vi "log analysis_gps.vi"() -> ()   [LabVIEW 2018] (continued)
\t1.658329\t-32.484656\t0.295000\t-0.002000\n\t\n15:23:55.0\tlog_raw\tgps_raw\t\tsystem status\tnormal 2 28.000000 0 0\trobot status\t288.054349\t67.318157\t10.021200\t0.546760\t1.689082\t-32.708365\t0.296000\t-0.003000\n\t\n15:23:55.5\tlog_raw\tgps_raw\t\tsystem status\tnormal 2 28.000000 0 0\trobot status\t288.169881\t67.229104\t10.024500\t0.591607\t1.733278\t-32.973827\t0.300000\t-0.009000\n\t\n15:23:56.1\tlog_raw\tgps_raw\t\tsystem status\tnormal 2 28.000000 0 0\trobot status\t288.285609\t67.140045\t10.028000\t0.529949\t1.703356\t-33.215106\t0.298000\t0.000000\n\t\n15:23:56.6\tlog_raw\tgps_raw\t\tsystem status\tnormal 2 28.000000 0 0\trobot status\t288.402896\t67.050197\t10.031000\t0.382545\t1.691064\t-33.405018\t0.303000\t-0.003000\n\t\n15:23:57.1\tlog_raw\tgps_raw\t\tsystem status\tnormal 2 28.100000 0 0\trobot status\t288.517996\t66.960392\t10.034600\t0.327686\t1.686813\t-33.520198\t0.306000\t0.000000\n\t\n15:23:57.6\tlog_raw\tgps_raw\t\tsystem status\tnormal 2 28.000000 0 0\trobot status\t288.617756\t66.878917\t10.037200\t0.388032\t1.762580\t-33.580696\t0.303000\t0.002000\n\t\n15:23:58.1\tlog_raw\tgps_raw\t\tsystem status\tnormal 2 28.000000 0 0\trobot status\t288.719206\t66.796540\t10.039700\t0.378367\t1.729293\t-33.611811\t0.296000\t-0.002000\n\t\n15:23:58.6\tlog_raw\tgps_raw\t\tsystem status\tnormal 2 28.000000 0 0\trobot status\t288.836366\t66.703108\t10.044100\t0.361317\t1.705497\t-33.618603\t0.298000\t0.013000\n\t\n15:23:59.1\tlog_raw\tgps_raw\t\tsystem status\tnormal 2 28.100000 0 0\trobot status\t288.954814\t66.609318\t10.047600\t0.188474\t1.632399\t-33.719352\t0.298000\t0.002000\n\t\n15:23:59.6\tlog_raw\tgps_raw\t\tsystem status\tnormal 2 28.100000 0 0\trobot status\t289.061981\t66.520928\t10.049900\t0.103210\t1.484384\t-33.752423\t0.295000\t0.002000\n\t\n15:24:00.1\tlog_raw\tgps_raw\t\tsystem status\tnormal 2 28.100000 0 0\trobot status\t289.171147\t66.430812\t10.051400\t0.015766\t1.445390\t-33.779693\t0.306000\t-0.012000\n\t\n15:24:00.6\tlog_raw\tgps_raw\t\tsystem status\tnormal 2 28.000000 0 0\trobot status\t289.280457\t66.339929\t10.054600\t-0.046571\t1.317193\t-33.648397\t0.286000\t0.023000\n\t\n15:24:01.1\tlog_raw\tgps_raw\t\tsystem status\tnormal 2 28.000000 0 0\trobot status\t289.389399\t66.249435\t10.057800\t-0.094988\t1.418269\t-33.490533\t0.253000\t0.072000\n\t\n15:24:01.6\tlog_raw\tgps_raw\t\tsystem status\tnormal 2 28.000000 0 0\trobot status\t289.499571\t66.160174\t10.062100\t-0.073967\t1.557073\t-33.178469\t0.257000\t0.075000\n\t\n15:24:02.1\tlog_raw\tgps_raw\t\tsystem status\tnormal 2 27.900000 0 0\trobot status\t289.611277\t66.070017\t10.066700\t-0.021080\t1.613738\t-32.746159\t0.225000\t0.126000\n\t\n15:24:02.6\tlog_raw\tgps_raw\t\tsystem status\tnormal 2 27.900000 0 0\trobot status\t289.725382\t65.979080\t10.070100\t-0.168702\t1.553048\t-32.226761\t0.295000\t0.028000\n\t\n15:24:03.1\tlog_raw\tgps_raw\t\tsystem status\tnormal 2 27.900000 0 0\trobot status\t289.838792\t65.888900\t10.073700\t-0.213673\t1.412012\t-31.737213\t0.429000\t-0.185000\n\t\n15:24:03.6\tlog_raw\tgps_raw\t#INSPVAXA,USB3,0,51.0,FINESTEERING,2107,282261.600,02008000,471d,15824;INS_ALIGNMENT_COMPLETE,INS_RTKFIXED,37.37072301964,126.72410864198,10.0789,22.3000,-0.1970,0.2354,0.0160,-0.160873741,1.322866529,121.119514583,0.4897,0.3148,0.6247,0.1298,0.1039,0.0767,0.1436,0.1490,5.0292,0f000001,0*85434b09\n\tsystem status\tnormal 2 27.900000 0 0\trobot status\t289.964535\t65.789209\t10.078900\t-0.160874\t1.322867\t-31.119515\t0.228000\t0.126000\n\t\n15:24:04.1\tlog_raw\tgps_raw\t#INSPVAXA,USB3,0,50.5,FINESTEERING,2107,282262.100,02008000,471d,15824;INS_ALIGNMENT_COMPLETE,INS_RTKFIXED,37.37072222272,126.72410992724,10.0823,22.3000,-0.1883,0.2369,0.0121,0.011480682,1.244674277,120.532236713,0.5693,0.3742,0.6825,0.1391,0.1098,0.0808,0.1445,0.1502,5.0254,0f000001,0*eae9fcde\n\tsystem status\tnormal 2 27.900000 0 0\trobot status\t290.078381\t65.700759\t10.082300\t0.011481\t1.244674\t-30.532237\t0.402000\t-0.130000\n\t\n15:24:04.6\tlog_raw\tgps_raw\t\tsystem status\tnormal 2 27.900000 0 0\trobot status\t290.181420\t65.629972\t10.084000\t-0.058152\t1.268255\t-30.033065\t0.380000\t-0.106000\n\t\n15:24:05.1\tlog_raw\tgps_raw\t\tsystem status\tnormal 2 27.900000 0 0\trobot status\t290.297225\t65.551573\t10.086000\t-0.219918\t1.150608\t-29.591429\t0.319000\t-0.025000\n\t\n15:24:05.6\tlog_raw\tgps_raw\t\tsystem status\tnormal 2 27.900000 0 0\trobot status\t290.413924\t65.470886\t10.089900\t-0.135917\t1.226255\t-29.162288\t0.353000\t-0.073000\n\t\n15:24:06.1\tlog_raw\tgps_raw\t\tsystem status\tnormal 2 28.000000 0 0\trobot status\t290.533106\t65.389467\t10.093600\t-0.089830\t1.183104\t-28.764617\t0.265000\t0.050000\n\t\n15:24:06.6\tlog_raw\tgps_raw\t\tsystem status\tnormal 2 28.000000 0 0\trobot status\t290.651382\t65.308209\t10.098300\t-0.148779\t1.341116\t-28.590743\t0.243000\t0.082000\n\t\n15:24:07.1\tlog_raw\tgps_raw\t\tsystem status\tnormal 2 28.000000 0 0\trobot status\t290.773116\t65.224624\t10.102200\t-0.235539\t1.356996\t-28.548470\t0.418000\t-0.171000\n\t\n15:24:07.6\tlog_raw\tgps_raw\t\tsystem status\tnormal 2 28.000000 0 0\trobot status\t290.891925\t65.142977\t10.104900\t-0.138580\t1.190893\t-28.503254\t0.342000\t-0.063000\n\t\n15:24:08.1\tlog_raw\tgps_raw\t\tsystem status\tnormal 2 28.000000 0 0\trobot status\t291.012059\t65.060352\t10.108400\t-0.108697\t1.088860\t-28.543618\t0.294000\t0.001000\n\t\n15:24:08.6\tlog_raw\tgps_raw\t#INSPVAXA,USB3,0,49.5,FINESTEERING,2107,282266.600,02000000,471d,15824;INS_ALIGNMENT_COMPLETE,INS_RTKFIXED,37.37071564001,126.72412194317,10.1142,22.3000,-0.1803,0.2485,0.0162,-0.167874326,0.987777383,118.589325472,0.4588,0.3004,0.5750,0.1240,0.0989,0.0769,0.1427,0.1481,5.0170,0f000001,0*94bf16e1\n\tsystem status\tnormal 2 28.000000 0 0\trobot status\t291.142733\t64.970143\t10.114200\t-0.167874\t0.987777\t-28.589325\t0.302000\t-0.008000\n\t\n15:24:09.1\tlog_raw\tgps_raw\t#INSPVAXA,USB3,0,51.5,FINESTEERING,2107,282267.100,02000000,471d,15824;INS_ALIGNMENT_COMPLETE,INS_RTKFIXED,37.37071488193,126.72412330620,10.1185,22.3000,-0.1782,0.2546,0.0105,-0.234897053,0.733993944,118.660329802,0.4588,0.3004,0.5750,0.1240,0.0989,0.0769,0.1427,0.1481,5.0170,0f000001,0*405246e9\n\tsystem status\tnormal 2 28.100000 0 0\trobot status\t291.263468\t64.886003\t10.118500\t-0.234897\t0.733994\t-28.660330\t0.301000\t-0.005000\n\t\n15:24:09.6\tlog_raw\tgps_raw\t\tsystem status\tnormal 2 28.100000 0 0\trobot status\t291.372920\t64.805007\t10.121900\t-0.262953\t0.652445\t-28.756882\t0.296000\t-0.023000\n\t\n15:24:10.1\tlog_raw\tgps_raw\t#INSPVAXA,USB3,0,50.5,FINESTEERING,2107,282268.100,02000000,471d,15824;INS_ALIGNMENT_COMPLETE,INS_RTKFIXED,37.37071326261,126.72412602696,10.1265,22.3000,-0.1797,0.2316,0.0106,-0.308837193,0.760008710,118.874107108,0.4588,0.3004,0.5750,0.1240,0.0989,0.0769,0.1427,0.1481,5.0170,0f000001,0*38424b3d\n\tsystem status\tnormal 2 28.100000 0 0\trobot status\t291.504468\t64.706275\t10.126500\t-0.308837\t0.760009\t-28.874107\t0.298000\t-0.019000\n\t\n15:24:10.6\tlog_raw\tgps_raw\t#INSPVAXA,USB3,0,50.5,FINESTEERING,2107,282268.600,02000000,471d,15824;INS_ALIGNMENT_COMPLETE,INS_RTKFIXED,37.37071245816,126.72412735967,10.1316,22.3000,-0.1815,0.2421,0.0127,-0.377106953,0.735852772,118.906106803,0.4588,0.3004,0.5750,0.1240,0.0989,0.0769,0.1427,0.1481,5.0170,0f000001,0*11ddd4c2\n\tsystem status\tnormal 2 28.100000 0 0\trobot status\t291.622517\t64.616989\t10.131600\t-0.377107\t0.735853\t-28.906107\t0.300000\t-0.012000\n\t\n15:24:11.1\tlog_raw\tgps_raw\t\tsystem status\tnormal 2 28.000000 0 0\trobot status\t291.731243\t64.535198\t10.136600\t-0.341882\t0.790169\t-29.060160\t0.298000\t-0.013000\n\t\n15:24:11.6\tlog_raw\tgps_raw\t#INSPVAXA,USB3,0,50.0,FINESTEERING,2107,282269.600,02000000,471d,15824;INS_ALIGNMENT_COMPLETE,INS_RTKFIXED,37.37071107493,126.72412999444,10.1387,22.3000,-0.1723,0.2314,0.0190,-0.521024846,1.079546483,119.280736819,0.5511,0.3672,0.6510,0.1337,0.1063,0.0814,0.1442,0.1496,5.0179,0f000001,0*5d398b6e\n\tsystem status\tnormal 2 28.100000 0 0\trobot status\t291.855901\t64.463464\t10.138700\t-0.521025\t1.079546\t-29.280737\t0.297000\t-0.008000\n\t\n15:24:12.1\tlog_raw\tgps_raw\t\tsystem status\tnormal 2 28.000000 0 0\trobot status\t291.955887\t64.404588\t10.140700\t-0.591155\t1.099206\t-29.528758\t0.294000\t-0.010000\n\t\n15:24:12.6\tlog_raw\tgps_raw\t#INSPVAXA,USB3,0,51.0,FINESTEERING,2107,282270.600,02008000,471d,15824;INS_ALIGNMENT_COMPLETE,INS_RTKFIXED,37.37070978971,126.72413254865,10.1460,22.3000,-0.1852,0.2381,0.0080,-0.437420088,1.249078779,119.796376349,0.5043,0.3305,0.6212,0.1261,0.1003,0.0792,0.1434,0.1486,5.0184,0f000001,0*9b5f8ba6\n\tsystem status\tnormal 2 28.000000 0 0\trobot status\t292.082149\t64.320817\t10.146000\t-0.437420\t1.249079\t-29.796376\t0.299000\t-0.013000\n\t\n15:24:13.1\tlog_raw\tgps_raw\t#INSPVAXA,USB3,0,47.5,FINESTEERING,2107,282271.100,02008000,471d,15824;INS_ALIGNMENT_COMPLETE,INS_RTKFIXED,37.37070909074,126.72413388392,10.1504,22.3000,-0.1800,0.2456,0.0054,-0.539837627,1.179431865,120.094630407,0.4787,0.3123,0.5991,0.1229,0.0985,0.0779,0.1432,0.1482,5.0193,0f000001,0*40acc907\n\tsystem status\tnormal 2 28.000000 0 0\trobot status\t292.200425\t64.243238\t10.150400\t-0.539838\t1.179432\t-30.094630\t0.297000\t-0.007000\n\t\n15:24:13.6\tlog_raw\tgps_raw\t#INSPVAXA,USB3,0,47.5,FINESTEERING,2107,282271.600,02008000,471d,15824;INS_ALIGNMENT_COMPLETE,INS_RTKFIXED,37.37070834780,126.72413522387,10.1531,22.3000,-0.1652,0.2443,0.0195,-0.572032410,1.056169102,120.353350938,0.4787,0.3123,0.5991,0.1229,0.0985,0.0779,0.1432,0.1482,5.0193,0f000001,0*1c071485\n\tsystem status\tnormal 2 28.000000 0 0\trobot status\t292.319115\t64.160778\t10.153100\t-0.572032\t1.056169\t-30.353351\t0.301000\t-0.020000\n\t\n15:24:14.1\tlog_raw\tgps_raw\t\tsystem status\tnormal 2 28.100000 0 0\trobot status\t292.425435\t64.085765\t10.154600\t-0.607784\t0.913539\t-30.523777\t0.299000\t-0.016000\n\t\n15:24:14.6\tlog_raw\tgps_raw\t#INSPVAXA,USB3,0,48.5,FINESTEERING,2107,282272.600,02008000,471d,15824;INS_ALIGNMENT_COMPLETE,INS_RTKFIXED,37.37070676202,126.72413789177,10.1597,22.3000,-0.1767,0.2382,0.0118,-0.374820510,0.656096150,120.799348362,0.4787,0.3123,0.5991,0.1229,0.0985,0.0779,0.1432,0.1482,5.0193,0f000001,0*9be2d9dc\n\tsystem status\tnormal 2 28.100000 0 0\trobot status\t292.555434\t63.984773\t10.159700\t-0.374821\t0.656096\t-30.799348\t0.293000\t-0.014000\n\t\n15:24:15.1\tlog_raw\tgps_raw\t\tsystem status\tnormal 2 28.000000 0 0\trobot status\t292.661239\t63.902459\t10.165100\t-0.316516\t0.670151\t-31.045836\t0.294000\t-0.010000\n\t\n15:24:15.6\tlog_raw\tgps_raw\t#INSPVAXA,USB3,0,51.5,FINESTEERING,2107,282273.600,02008000,471d,15824;INS_ALIGNMENT_COMPLETE,INS_RTKFIXED,37.37070511778,126.72414055042,10.1715,22.3000,-0.1870,0.2363,0.0134,-0.459769985,0.798437213,121.336357877,0.4787,0.3123,0.5991,0.1229,0.0985,0.0779,0.1432,0.1482,5.0193,0f000001,0*703348aa\n\tsystem status\tnormal 2 28.000000 0 0\trobot status\t292.790932\t63.802279\t10.171500\t-0.459770\t0.798437\t-31.336358\t0.297000\t-0.009000\n\t\n15:24:16.1\tlog_raw\tgps_raw\t\tsystem status\tnormal 2 28.100000 0 0\trobot status\t292.895056\t63.721026\t10.176300\t-0.551373\t0.887898\t-31.600267\t0.298000\t-0.009000\n\t\n15:24:16.6\tlog_raw\tgps_raw\t#INSPVAXA,USB3,0,50.0,FINESTEERING,2107,282274.600,02000000,471d,15824;INS_ALIGNMENT_COMPLETE,INS_RTKFIXED,37.37070363879,126.72414308570,10.1749,22.3000,-0.1813,0.2312,0.0078,-0.604469553,1.084486216,121.923542581,0.5575,0.3692,0.6704,0.1333,0.1077,0.0814,0.1446,0.1496,5.0225,0f000001,0*5c099128\n\tsystem status\tnormal 2 28.100000 0 0\trobot status\t293.015503\t63.638127\t10.174900\t-0.604470\t1.084486\t-31.923543\t0.297000\t-0.006000\n\t\n15:24:17.1\tlog_raw\tgps_raw\t#INSPVAXA,USB3,0,50.5,FINESTEERING,2107,282275.100,02000000,471d,15824;INS_ALIGNMENT_COMPLETE,INS_RTKFIXED,37.37070296140,126.72414429321,10.1745,22.3000,-0.1748,0.2312,0.0107,-0.634765121,1.047187447,122.187120855,0.5046,0.3310,0.6337,0.1261,0.1021,0.0787,0.1438,0.1486,5.0224,0f000001,0*d0387721\n\tsystem status\tnormal 2 28.100000 0 0\trobot status\t293.122463\t63.562943\t10.174500\t-0.634765\t1.047187\t-32.187121\t0.299000\t-0.006000\n\t\n15:24:17.6\tlog_raw\tgps_raw\t#INSPVAXA,USB3,0,50.5,FINESTEERING,2107,282275.600,02000000,471d,15824;INS_ALIGNMENT_COMPLETE,INS_RTKFIXED,37.37070222382,126.72414554188,10.1759,22.3000,-0.1770,0.2216,0.0167,-0.613341338,0.949181726,122.390549431,0.5046,0.3310,0.6337,0.1261,0.1021,0.0787,0.1438,0.1486,5.0224,0f000001,0*c2bde323\n\tsystem status\tnormal 2 28.000000 0 0\trobot status\t293.233068\t63.481079\t10.175900\t-0.613341\t0.949182\t-32.390549\t0.296000\t-0.002000\n\t\n15:24:18.1\tlog_raw\tgps_raw\t#INSPVAXA,USB3,0,49.0,FINESTEERING,2107,282276.100,02000000,471d,15824;INS_ALIGNMENT_COMPLETE,INS_RTKFIXED,37.37070146570,126.72414680907,10.1773,22.3000,-0.1774,0.2243,0.0157,-0.609174519,0.899706635,122.569585175,0.4767,0.3125,0.6072,0.1235,0.1004,0.0773,0.1434,0.1482,5.0223,0f000001,0*a35fb81b\n\tsystem status\tnormal 2 28.100000 0 0\trobot status\t293.345313\t63.396935\t10.177300\t-0.609175\t0.899707\t-32.569585\t0.299000\t0.000000\n\t\n15:24:18.6\tlog_raw\tgps_raw\t\tsystem status\tnormal 2 28.100000 0 0\trobot status\t293.444232\t63.320197\t10.180300\t-0.593656\t0.818984\t-32.795506\t0.301000\t-0.003000\n\t\n15:24:19.1\tlog_raw\tgps_raw\t#INSPVAXA,USB3,0,50.0,FINESTEERING,2107,282277.100,02000000,471d,15824;INS_ALIGNMENT_COMPLETE,INS_RTKFIXED,37.37069991504,126.72414929974,10.1840,22.3000,-0.1767,0.2226,0.0047,-0.557997930,0.665249909,123.001928540,0.4767,0.3125,0.6072,0.1235,0.1004,0.0773,0.1434,0.1482,5.0223,0f000001,0*cb3103e7\n\tsystem status\tnormal 2 28.100000 0 0\trobot status\t293.565933\t63.224828\t10.184000\t-0.557998\t0.665250\t-33.001929\t0.296000\t0.002000\n\t\n15:24:19.6\tlog_raw\tgps_raw\t\tsystem status\tnormal 2 28.100000 0 0\trobot status\t293.665372\t63.142839\t10.189000\t-0.617323\t0.688216\t-33.148551\t0.293000\t0.009000\n\t\n15:24:20.1\tlog_raw\tgps_raw\t#INSPVAXA,USB3,0,53.0,FINESTEERING,2107,282278.100,02000000,471d,15824;INS_ALIGNMENT_COMPLETE,INS_RTKFIXED,37.37069823681,126.72415183772,10.1961,22.3000,-0.1823,0.2204,0.0074,-0.523658025,0.566082067,123.287197308,0.4767,0.3125,0.6072,0.1235,0.1004,0.0773,0.1434,0.1482,5.0223,0f000001,0*25d51a4b\n\tsystem status\tnormal 2 28.100000 0 0\trobot status\t293.790743\t63.038563\t10.196100\t-0.523658\t0.566082\t-33.287197\t0.303000\t-0.002000\n\t\n15:24:20.6\tlog_raw\tgps_raw\t\tsystem status\tnormal 2 28.100000 0 0\trobot status\t293.892481\t62.953714\t10.201200\t-0.497645\t0.480961\t-33.302974\t0.300000\t0.011000\n\t\n15:24:21.1\tlog_raw\tgps_raw\t\tsystem status\tnormal 2 28.100000 0 0\trobot status\t294.010445\t62.857710\t10.205900\t-0.584538\t0.459280\t-33.393453\t0.299000\t0.008000\n\t\n15:24:21.6\tlog_raw\tgps_raw\t\tsystem status\tnormal 2 28.100000 0 0\trobot status\t294.125019\t62.772862\t10.206400\t-0.680267\t0.496944\t-33.443344\t0.303000\t0.004000\n\t\n15:24:22.1\tlog_raw\tgps_raw\t#INSPVAXA,USB3,0,47.5,FINESTEERING,2107,282280.100,02000000,471d,15824;INS_ALIGNMENT_COMPLETE,INS_RTKFIXED,37.37069498335,126.72415703248,10.2090,22.3000,-0.1979,0.2492,0.0153,-0.691574925,0.436072461,123.457665548,0.5547,0.3701,0.6738,0.1343,0.1087,0.0808,0.1445,0.1496,5.0239,0f000001,0*1cc0a1a6\n\tsystem status\tnormal 2 28.100000 0 0\trobot status\t294.250886\t62.677463\t10.209000\t-0.691575\t0.436072\t-33.457666\t0.308000\t0.006000\n\t\n15:24:22.6\tlog_raw\tgps_raw\t\tsystem status\tnormal 2 28.000000 0 0\trobot status\t294.357425\t62.588733\t10.214300\t-0.468577\t0.095903\t-33.413871\t0.285000\t0.024000\n\t\n15:24:23.1\tlog_raw\tgps_raw\t#INSPVAXA,USB3,0,49.5,FINESTEERING,2107,282281.100,02000000,471d,15824;INS_ALIGNMENT_COMPLETE,INS_RTKFIXED,37.37069324003,126.72415967576,10.2193,22.3000,-0.1883,0.2410,0.0110,-0.444587067,-0.239892052,123.232720595,0.5547,0.3701,0.6738,0.1343,0.1087,0.0808,0.1445,0.1496,5.0239,0f000001,0*fc1f5c5f\n\tsystem status\tnormal 2 28.000000 0 0\trobot status\t294.485024\t62.483973\t10.219300\t-0.444587\t-0.239892\t-33.232721\t0.336000\t-0.039000\n\t\n15:24:23.6\tlog_raw\tgps_raw\t\tsystem status\tnormal 2 28.000000 0 0\trobot status\t294.590664\t62.401031\t10.222200\t-0.677387\t-0.510813\t-32.931277\t0.345000\t-0.055000\n\t\n15:24:24.1\tlog_raw\tgps_raw\t#INSPVAXA,USB3,0,47.5,FINESTEERING,2107,282282.100,02000000,471d,15824;INS_ALIGNMENT_COMPLETE,INS_RTKFIXED,37.37069160850,126.72416229361,10.2264,22.3000,-0.1858,0.2281,-0.0001,-0.736056303,-0.906540815,122.497361054,0.5875,0.3887,0.7203,0.1380,0.1105,0.0818,0.1447,0.1498,5.0279,0f000001,0*0c5128b7\n\tsystem status\tnormal 2 28.000000 0 0\trobot status\t294.716909\t62.302890\t10.226400\t-0.736056\t-0.906541\t-32.497361\t0.314000\t-0.011000\n\t\n15:24:24.6\tlog_raw\tgps_raw\t#INSPVAXA,USB3,0,47.5,FINESTEERING,2107,282282.600,02000000,471d,15824;INS_ALIGNMENT_COMPLETE,INS_RTKFIXED,37.37069089697,126.72416351730,10.2196,22.3000,-0.1871,0.2326,0.0042,-0.425257190,-0.862348838,121.960644857,0.5875,0.3887,0.7203,0.1380,0.1105,0.0818,0.1447,0.1498,5.0279,0f000001,0*490a0fa5\n\tsystem status\tnormal 2 27.900000 0 0\trobot status\t294.825301\t62.223917\t10.219600\t-0.425257\t-0.862349\t-31.960645\t0.346000\t-0.056000\n\t\n15:24:25.1\tlog_raw\tgps_raw\t\tsystem status\tnormal 2 27.900000 0 0\trobot status\t294.924203\t62.153574\t10.212800\t-0.190843\t-0.823864\t-31.404317\t0.359000\t-0.071000\n\t\n15:24:25.6\tlog_raw\tgps_raw\t#INSPVAXA,USB3,0,46.5,FINESTEERING,2107,282283.600,02008000,471d,15824;INS_ALIGNMENT_COMPLETE,INS_RTKFIXED,37.37068940958,126.72416607579,10.2138,22.3000,-0.1636,0.2189,-0.0003,-0.120036604,-0.860841459,120.892387916,0.5875,0.3887,0.7203,0.1380,0.1105,0.0818,0.1447,0.1498,5.0279,0f000001,0*9192f1a2\n\tsystem status\tnormal 2 27.900000 0 0\trobot status\t295.051928\t62.058832\t10.213800\t-0.120037\t-0.860841\t-30.892388\t0.401000\t-0.149000\n\t\n15:24:26.1\tlog_raw\tgps_raw\t#INSPVAXA,USB3,0,51.5,FINESTEERING,2107,282284.100,02008000,471d,15824;INS_ALIGNMENT_COMPLETE,INS_RTKFIXED,37.37068864878,126.72416738015,10.2177,22.3000,-0.1641,0.2313,0.0038,-0.033754752,-0.589658100,120.436095799,0.5875,0.3887,0.7203,0.1380,0.1105,0.0818,0.1447,0.1498,5.0279,0f000001,0*0148cd2e\n\tsystem status\tnormal 2 27.900000 0 0\trobot status\t295.167466\t61.974391\t10.217700\t-0.033755\t-0.589658\t-30.436096\t0.215000\t0.132000\n\t\n15:24:26.6\tlog_raw\tgps_raw\t#INSPVAXA,USB3,0,51.5,FINESTEERING,2107,282284.600,02008000,471d,15824;INS_ALIGNMENT_COMPLETE,INS_RTKFIXED,37.37068791248,126.72416871170,10.2207,22.3000,-0.1613,0.2366,0.0105,-0.227472838,-0.490349868,119.960742273,0.5875,0.3887,0.7203,0.1380,0.1105,0.0818,0.1447,0.1498,5.0279,0f000001,0*af559696\n\tsystem status\tnormal 2 27.900000 0 0\trobot status\t295.285413\t61.892668\t10.220700\t-0.227473\t-0.490350\t-29.960742\t0.213000\t0.142000\n\t\n15:24:27.1\tlog_raw\tgps_raw\t#INSPVAXA,USB3,0,51.5,FINESTEERING,2107,282285.100,02008000,471d,15824;INS_ALIGNMENT_COMPLETE,INS_RTKFIXED,37.37068720846,126.72417000092,10.2252,22.3000,-0.1602,0.2440,0.0066,-0.187971792,0.385088793,119.635511852,0.5949,0.3921,0.7470,0.1392,0.1132,0.0817,0.1449,0.1501,5.0298,0f000001,0*026b0f4f\n\tsystem status\tnormal 2 27.900000 0 0\trobot status\t295.399609\t61.814529\t10.225200\t-0.187972\t0.385089\t-29.635512\t0.333000\t-0.021000\n\t\n15:24:27.6\tlog_raw\tgps_raw\t#INSPVAXA,USB3,0,52.0,FINESTEERING,2107,282285.600,02008000,471d,15824;INS_ALIGNMENT_COMPLETE,INS_RTKFIXED,37.37068652184,126.72417128801,10.2137,22.3000,-0.1658,0.2472,-0.0117,-0.055492896,0.657869792,119.429156162,0.5949,0.3921,0.7470,0.1392,0.1132,0.0817,0.1449,0.1501,5.0298,0f000001,0*cfd09dcb\n\tsystem status\tnormal 2 28.000000 0 0\trobot status\t295.513618\t61.738321\t10.213700\t-0.055493\t0.657870\t-29.429156\t0.222000\t0.118000\n\t\n15:24:28.1\tlog_raw\tgps_raw\t#INSPVAXA,USB3,0,48.5,FINESTEERING,2107,282286.100,02008000,471d,15824;INS_ALIGNMENT_COMPLETE,INS_RTKFIXED,37.37068585553,126.72417255759,10.2052,22.3000,-0.1551,0.2284,0.0107,-0.089152312,0.639970928,119.250576511,0.5190,0.3392,0.6809,0.1320,0.1082,0.0780,0.1441,0.1491,5.0307,0f000001,0*ec53885d\n\tsystem status\tnormal 2 28.000000 0 0\trobot status\t295.626075\t61.664367\t10.205200\t-0.089152\t0.639971\t-29.250577\t0.247000\t0.053000\n\t\n15:24:28.6\tlog_raw\tgps_raw\t#INSPVAXA,USB3,0,48.5,FINESTEERING,2107,282286.600,02008000,471d,15824;INS_ALIGNMENT_COMPLETE,INS_RTKFIXED,37.37068514150,126.72417389818,10.2001,22.3000,-0.1412,0.2197,0.0066,0.024364093,0.832001131,119.298455875,0.5190,0.3392,0.6809,0.1320,0.1082,0.0780,0.1441,0.1491,5.0307,0f000001,0*de9bf723\n\tsystem status\tnormal 2 28.100000 0 0\trobot status\t295.744822\t61.585116\t10.200100\t0.024364\t0.832001\t-29.298456\t0.272000\t0.056000\n\t\n15:24:29.1\tlog_raw\tgps_raw\t#INSPVAXA,USB3,0,48.5,FINESTEERING,2107,282287.100,02008000,471d,15824;INS_ALIGNMENT_COMPLETE,INS_RTKFIXED,37.37068448744,126.72417519191,10.1977,22.3000,-0.1331,0.1859,0.0151,-0.327488179,0.840633219,119.294501197,0.4827,0.3161,0.6365,0.1297,0.1073,0.0763,0.1436,0.1487,5.0297,0f000001,0*ec0356ba\n\tsystem status\tnormal 2 28.100000 0 0\trobot status\t295.859419\t61.512521\t10.197700\t-0.327488\t0.840633\t-29.294501\t0.273000\t-0.012000\n\t\n15:24:29.6\tlog_raw\tgps_raw\t#INSPVAXA,USB3,0,49.5,FINESTEERING,2107,282287.600,02000000,471d,15824;INS_ALIGNMENT_COMPLETE,INS_RTKFIXED,37.37068376486,126.72417656780,10.2009,22.3000,-0.1622,0.2304,0.0144,-0.264314636,1.151154189,119.357397918,0.4827,0.3161,0.6365,0.1297,0.1073,0.0763,0.1436,0.1487,5.0297,0f000001,0*1ac61951\n\tsystem status\tnormal 2 28.000000 0 0\trobot status\t295.981293\t61.432322\t10.200900\t-0.264315\t1.151154\t-29.357398\t0.309000\t0.000000\n\t\n15:24:30.1\tlog_raw\tgps_raw\t#INSPVAXA,USB3,0,52.0,FINESTEERING,2107,282288.100,02000000,471d,15824;INS_ALIGNMENT_COMPLETE,INS_RTKFIXED,37.37068313188,126.72417778864,10.2013,22.3000,-0.1464,0.2451,0.0101,-0.437974736,2.271326824,119.414001695,0.4827,0.3161,0.6365,0.1297,0.1073,0.0763,0.1436,0.1487,5.0297,0f000001,0*f8a30918\n\tsystem status\tnormal 2 28.000000 0 0\trobot status\t296.089433\t61.362067\t10.201300\t-0.437975\t2.271327\t-29.414002\t0.304000\t-0.003000\n\t\n15:24:30.6\tlog_raw\tgps_raw\t#INSPVAXA,USB3,0,52.0,FINESTEERING,2107,282288.600,02000000,471d,15824;INS_ALIGNMENT_COMPLETE,INS_RTKFIXED,37.37068248207,126.72417903271,10.2071,22.3000,-0.1554,0.2479,0.0102,-0.520482478,3.090095843,119.464562963,0.4827,0.3161,0.6365,0.1297,0.1073,0.0763,0.1436,0.1487,5.0297,0f000001,0*4436d63b\n\tsystem status\tnormal 2 28.000000 0 0\trobot status\t296.199631\t61.289944\t10.207100\t-0.520482\t3.090096\t-29.464563\t0.306000\t-0.003000\n\t\n15:24:31.1\tlog_raw\tgps_raw\t#INSPVAXA,USB3,0,48.0,FINESTEERING,2107,282289.100,02000000,471d,15824;INS_ALIGNMENT_COMPLETE,INS_RTKFIXED,37.37068179402,126.72418031784,10.2124,22.3000,-0.1466,0.2345,0.0076,-0.435594765,3.881928783,119.627439178,0.5155,0.3438,0.6451,0.1390,0.1110,0.0782,0.1436,0.1489,5.0203,0f000001,0*d705b298\n\tsystem status\tnormal 2 28.000000 0 0\trobot status\t296.313465\t61.213577\t10.212400\t-0.435595\t3.881929\t-29.627439\t0.294000\t-0.019000\n\t\n15:24:31.6\tlog_raw\tgps_raw\t#INSPVAXA,USB3,0,48.0,FINESTEERING,2107,282289.600,02000000,471d,15824;INS_ALIGNMENT_COMPLETE,INS_RTKFIXED,37.37068106233,126.72418156036,10.2167,22.3000,-0.1573,0.2453,0.0197,-0.196955820,4.346907241,119.830177459,0.5155,0.3438,0.6451,0.1390,0.1110,0.0782,0.1436,0.1489,5.0203,0f000001,0*c638875e\n\tsystem status\tnormal 2 28.000000 0 0\trobot status\t296.423526\t61.132367\t10.216700\t-0.196956\t4.346907\t-29.830177\t0.300000\t-0.016000\n\t\n15:24:32.1\tlog_raw\tgps_raw\t#INSPVAXA,USB3,0,45.0,FINESTEERING,2107,282290.100,02000000,471d,15824;INS_ALIGNMENT_COMPLETE,INS_RTKFIXED,37.37068031183,126.72418287504,10.2233,22.3000,-0.1663,0.2481,0.0180,-0.098835981,4.376797831,120.158403122,0.5155,0.3438,0.6451,0.1390,0.1110,0.0782,0.1436,0.1489,5.0203,0f000001,0*f931a41f\n\tsystem status\tnormal 2 28.000000 0 0\trobot status\t296.539978\t61.049069\t10.223300\t-0.098836\t4.376798\t-30.158403\t0.298000\t-0.016000\n\t\n15:24:32.6\tlog_raw\tgps_raw\t#INSPVAXA,USB3,0,45.0,FINESTEERING,2107,282290.600,02000000,471d,15824;INS_ALIGNMENT_COMPLETE,INS_RTKFIXED,37.37067956238,126.72418428483,10.2337,22.3000,-0.1707,0.2482,0.0265,-0.202932482,4.159469739,120.506147685,0.5155,0.3438,0.6451,0.1390,0.1110,0.0782,0.1436,0.1489,5.0203,0f000001,0*908c714d\n\tsystem status\tnormal 2 28.000000 0 0\trobot status\t296.664855\t60.965887\t10.233700\t-0.202932\t4.159470\t-30.506148\t0.300000\t-0.025000\n\t\n15:24:33.1\tlog_raw\tgps_raw\t#INSPVAXA,USB3,0,45.0,FINESTEERING,2107,282291.100,02000000,471d,15824;INS_ALIGNMENT_COMPLETE,INS_RTKFIXED,37.37067879937,126.72418567734,10.2444,22.3000,-0.1651,0.2543,0.0207,-0.251060851,3.844476935,120.878401990,0.5409,0.3575,0.6537,0.1355,0.1073,0.0795,0.1434,0.1485,4.9849,0f000001,0*d6642fae\n\tsystem status\tnormal 2 28.000000 0 0\trobot status\t296.788201\t60.881200\t10.244400\t-0.251061\t3.844477\t-30.878402\t0.299000\t-0.019000\n\t\n15:24:33.6\tlog_raw\tgps_raw\t#INSPVAXA,USB3,0,49.0,FINESTEERING,2107,282291.600,02000000,471d,15824;INS_ALIGNMENT_COMPLETE,INS_RTKFIXED,37.37067799408,126.72418700521,10.2537,22.3000,-0.1763,0.2581,0.0156,-0.182414041,3.404030284,121.216304080,0.5409,0.3575,0.6537,0.1355,0.1073,0.0795,0.1434,0.1485,4.9849,0f000001,0*0bbc7934\n\tsystem status\tnormal 2 28.000000 0 0\trobot status\t296.905822\t60.791821\t10.253700\t-0.182414\t3.404030\t-31.216304\t0.300000\t-0.019000\n\t\n15:24:34.1\tlog_raw\tgps_raw\t#INSPVAXA,USB3,0,45.5,FINESTEERING,2107,282292.100,02000000,471d,15824;INS_ALIGNMENT_COMPLETE,INS_RTKFIXED,37.37067717574,126.72418831770,10.2613,22.3000,-0.1798,0.2515,0.0164,-0.016177386,3.020104731,121.543147805,0.5007,0.3269,0.6199,0.1278,0.1011,0.0781,0.1427,0.1475,4.9679,0f000001,0*266eeccf\n\tsystem status\tnormal 2 28.000000 0 0\trobot status\t297.022080\t60.700994\t10.261300\t-0.016177\t3.020105\t-31.543148\t0.290000\t-0.026000\n\t\n15:24:34.6\tlog_raw\tgps_raw\t#INSPVAXA,USB3,0,45.5,FINESTEERING,2107,282292.600,02000000,471d,15824;INS_ALIGNMENT_COMPLETE,INS_RTKFIXED,37.37067636900,126.72418961762,10.2690,22.3000,-0.1769,0.2534,0.0080,-0.042843128,2.826759878,121.907768191,0.5007,0.3269,0.6199,0.1278,0.1011,0.0781,0.1427,0.1475,4.9679,0f000001,0*aaae4f23\n\tsystem status\tnormal 2 28.000000 0 0\trobot status\t297.137225\t60.611454\t10.269000\t-0.042843\t2.826760\t-31.907768\t0.292000\t-0.018000\n\t\n15:24:35.1\tlog_raw\tgps_raw\t#INSPVAXA,USB3,0,45.5,FINESTEERING,2107,282293.100,02000000,471d,15824;INS_ALIGNMENT_COMPLETE,INS_RTKFIXED,37.37067553892,126.72419093232,10.2760,22.3000,-0.1811,0.2495,0.0116,-0.008430473,2.413814082,122.277222921,0.4766,0.3108,0.5954,0.1241,0.0990,0.0774,0.1425,0.1470,4.9617,0f000001,0*c888aeda\n\tsystem status\tnormal 2 28.000000 0 0\trobot status\t297.253679\t60.519324\t10.276000\t-0.008430\t2.413814\t-32.277223\t0.308000\t-0.003000\n\t\n15:24:35.6\tlog_raw\tgps_raw\t#INSPVAXA,USB3,0,46.5,FINESTEERING,2107,282293.600,02000000,471d,15824;INS_ALIGNMENT_COMPLETE,INS_RTKFIXED,37.37067472793,126.72419224415,10.2820,22.3000,-0.1803,0.2324,0.0113,-0.180884788,2.125088791,122.585479065,0.4766,0.3108,0.5954,0.1241,0.0990,0.0774,0.1425,0.1470,4.9617,0f000001,0*8a54f30e\n\tsystem status\tnormal 2 28.000000 0 0\trobot status\t297.369878\t60.429312\t10.282000\t-0.180885\t2.125089\t-32.585479\t0.274000\t-0.042000\n\t\n15:24:36.1\tlog_raw\tgps_raw\t#INSPVAXA,USB3,0,46.5,FINESTEERING,2107,282294.100,02008000,471d,15824;INS_ALIGNMENT_COMPLETE,INS_RTKFIXED,37.37067392240,126.72419354245,10.2863,22.3000,-0.1909,0.2309,0.0096,-0.404437997,1.924119291,122.825127987,0.4614,0.3022,0.5776,0.1224,0.0977,0.0772,0.1423,0.1468,4.9609,0f000001,0*f2faedc4\n\tsystem status\tnormal 2 28.000000 0 0\trobot status\t297.484880\t60.339907\t10.286300\t-0.404438\t1.924119\t-32.825128\t0.293000\t-0.008000\n\t\n15:24:36.6\tlog_raw\tgps_raw\t#DUALANTENNAHEADINGA,USB3,0,47.0,FINESTEERING,2107,282294.600,02008000,d426,15824;SOL_COMPUTED,NARROW_FLOAT,-1.000000000,121.189437866,-60.258087158,0.0,360.000000000,180.000000000,\"631T\",18,7,7,5,04,00,20,03*d581effc\n\tsystem status\tnormal 2 28.100000 0 0\trobot status\t297.596477\t60.250156\t10.290000\t-0.474567\t1.563892\t-33.134759\t0.291000\t0.000000\n\t\n15:24:37.1\tlog_raw\tgps_raw\t#DUALANTENNAHEADINGA,USB3,0,45.0,FINESTEERING,2107,282295.100,02008000,d426,15824;SOL_COMPUTED,L1_FLOAT,-1.000000000,102.362266541,-42.452087402,0.0,360.000000000,180.000000000,\"631T\",17,6,6,3,04,00,20,01*c6a3d1e1\n\tsystem status\tnormal 2 28.000000 0 0\trobot status\t297.709107\t60.159225\t10.294100\t-0.608566\t1.421142\t-33.394057\t0.298000\t-0.001000\n\t\n15:24:37.6\tlog_raw\tgps_raw\t#DUALANTENNAHEADINGA,USB3,0,45.0,FINESTEERING,2107,282295.600,02008000,d426,15824;SOL_COMPUTED,L1_FLOAT,-1.000000000,103.041458130,-42.702667236,0.0,360.000000000,180.000000000,\"631T\",15,6,6,3,04,00,20,01*07943439\n\tsystem status\tnormal 2 28.100000 0 0\trobot status\t297.819501\t60.068897\t10.297700\t-0.835461\t1.405990\t-33.622422\t0.297000\t0.001000\n\t\n15:24:38.1\tlog_raw\tgps_raw\t#INSPVAXA,USB3,0,45.5,FINESTEERING,2107,282296.100,02008000,471d,15824;INS_ALIGNMENT_COMPLETE,INS_RTKFIXED,37.37067068708,126.72419852812,10.3007,22.3000,-0.1831,0.2265,0.0055,-1.180023346,1.380731558,123.921580343,0.4463,0.2958,0.5559,0.1206,0.0957,0.0774,0.1421,0.1465,4.9614,0f000001,0*6538f2e2\n\tsystem status\tnormal 2 28.100000 0 0\trobot status\t297.926502\t59.980821\t10.300700\t-1.180023\t1.380732\t-33.921580\t0.296000\t0.006000\n\t\n15:24:38.6\tlog_raw\tgps_raw\t#DUALANTENNAHEADINGA,USB3,0,45.5,FINESTEERING,2107,282296.600,02008000,d426,15824;INSUFFICIENT_OBS,NONE,0.000000000,0.000000000,0.000000000,0.0,0.000000000,0.000000000,\"\",0,0,0,0,00,00,00,00*630506ca\n\tsystem status\tnormal 2 28.000000 0 0\trobot status\t298.030524\t59.893999\t10.304700\t-1.378362\t1.706847\t-34.188339\t0.296000\t0.003000\n\t\n15:24:39.1\tlog_raw\tgps_raw\t#INSPVAXA,USB3,0,50.5,FINESTEERING,2107,282297.100,02008000,471d,15824;INS_ALIGNMENT_COMPLETE,INS_RTKFIXED,37.37066909241,126.72420090990,10.3083,22.3000,-0.1861,0.2064,0.0054,-1.451232970,2.139492751,124.282872789,0.4463,0.2958,0.5559,0.1206,0.0957,0.0774,0.1421,0.1465,4.9614,0f000001,0*92259f00\n\tsystem status\tnormal 2 28.000000 0 0\trobot status\t298.137476\t59.803829\t10.308300\t-1.451233\t2.139493\t-34.282873\t0.292000\t0.000000\n\t\n15:24:39.6\tlog_raw\tgps_raw\t#INSPVAXA,USB3,0,50.5,FINESTEERING,2107,282297.600,02008000,471d,15824;INS_ALIGNMENT_COMPLETE,INS_RTKFIXED,37.37066824319,126.72420217982,10.3132,22.3000,-0.1844,0.2206,0.0132,-1.291295595,2.299474120,124.306238371,0.4463,0.2958,0.5559,0.1206,0.0957,0.0774,0.1421,0.1465,4.9614,0f000001,0*08710687\n\tsystem status\tnormal 2 28.000000 0 0\trobot status\t298.249964\t59.709575\t10.313200\t-1.291296\t2.299474\t-34.306238\t0.298000\t0.017000\n\t\n15:24:40.1\tlog_raw\tgps_raw\t#INSPVAXA,USB3,0,47.5,FINESTEERING,2107,282298.100,02000000,471d,15824;INS_ALIGNMENT_COMPLETE,INS_RTKFIXED,37.37066736588,126.72420348765,10.3177,22.3000,-0.2044,0.2368,0.0054,-0.934530380,2.484268060,124.268578123,0.4463,0.2958,0.5559,0.1206,0.0957,0.0774,0.1421,0.1465,4.9614,0f000001,0*e22edcc5\n\tsystem status\tnormal 2 28.000000 0 0\trobot status\t298.365809\t59.612203\t10.317700\t-0.934530\t2.484268\t-34.268578\t0.304000\t0.018000\n\t\n15:24:40.6\tlog_raw\tgps_raw\t#INSPVAXA,USB3,0,47.5,FINESTEERING,2107,282298.600,02000000,471d,15824;INS_ALIGNMENT_COMPLETE,INS_RTKFIXED,37.37066650414,126.72420478717,10.3223,22.3000,-0.2012,0.2369,0.0184,-0.644074301,2.480545222,124.200345870,0.4463,0.2958,0.5559,0.1206,0.0957,0.0774,0.1421,0.1465,4.9614,0f000001,0*352785c6\n\tsystem status\tnormal 2 28.000000 0 0\trobot status\t298.480919\t59.516559\t10.322300\t-0.644074\t2.480545\t-34.200346\t0.295000\t0.023000\n\t\n15:24:41.1\tlog_raw\tgps_raw\t#DUALANTENNAHEADINGA,USB3,0,47.5,FINESTEERING,2107,282299.100,02000000,d426,15824;SOL_COMPUTED,L1_FLOAT,-1.000000000,104.413963318,-39.969207764,0.0,360.000000000,180.000000000,\"631T\",13,6,6,3,04,00,20,01*0865e994\n\tsystem status\tnormal 2 28.000000 0 0\trobot status\t298.596655\t59.422581\t10.327500\t-0.520458\t2.566476\t-34.126237\t0.285000\t0.036000\n\t\n15:24:41.6\tlog_raw\tgps_raw\t#INSPVAXA,USB3,0,50.5,FINESTEERING,2107,282299.600,02000000,471d,15824;INS_ALIGNMENT_COMPLETE,INS_RTKFIXED,37.37066485429,126.72420728055,10.3338,22.3000,-0.1766,0.2255,0.0106,-0.427425360,2.613001308,123.918175159,0.5467,0.3647,0.6429,0.1311,0.1043,0.0822,0.1440,0.1485,4.9572,0f000001,0*9195cd30\n\tsystem status\tnormal 2 28.000000 0 0\trobot status\t298.701778\t59.333443\t10.333800\t-0.427425\t2.613001\t-33.918175\t0.388000\t-0.119000\n\t\n15:24:42.1\tlog_raw\tgps_raw\t#DUALANTENNAHEADINGA,USB3,0,48.5,FINESTEERING,2107,282300.100,02000000,d426,15824;INSUFFICIENT_OBS,NONE,0.000000000,0.000000000,0.000000000,0.0,0.000000000,0.000000000,\"\",0,0,0,0,00,00,00,00*e37ee9dd\n\tsystem status\tnormal 2 27.900000 0 0\trobot status\t298.802912\t59.246374\t10.341300\t0.030100\t2.603217\t-33.349741\t0.317000\t-0.005000\n\t\n15:24:42.6\tlog_raw\tgps_raw\t#INSPVAXA,USB3,0,48.5,FINESTEERING,2107,282300.600,02000000,471d,15824;INS_ALIGNMENT_COMPLETE,INS_RTKFIXED,37.37066328709,126.72420961412,10.3498,22.3000,-0.1736,0.2244,0.0088,0.359177910,2.809986470,122.746384248,0.5045,0.3294,0.6194,0.1239,0.0993,0.0801,0.1433,0.1477,4.9538,0f000001,0*bd968cc8\n\tsystem status\tnormal 2 27.900000 0 0\trobot status\t298.908482\t59.159501\t10.349800\t0.359178\t2.809986\t-32.746384\t0.347000\t-0.031000\n\t\n15:24:43.1\tlog_raw\tgps_raw\t#INSPVAXA,USB3,0,49.0,FINESTEERING,2107,282301.100,02000000,471d,15824;INS_ALIGNMENT_COMPLETE,INS_RTKFIXED,37.37066253151,126.72421082792,10.3582,22.3000,-0.1761,0.2216,0.0197,0.484810078,3.068722182,122.157081229,0.5045,0.3294,0.6194,0.1239,0.0993,0.0801,0.1433,0.1477,4.9538,0f000001,0*fc57e6fe\n\tsystem status\tnormal 2 27.900000 0 0\trobot status\t299.015998\t59.075639\t10.358200\t0.484810\t3.068722\t-32.157081\t0.218000\t0.155000\n\t\n15:24:43.6\tlog_raw\tgps_raw\t#DUALANTENNAHEADINGA,USB3,0,49.0,FINESTEERING,2107,282301.600,02000000,d426,15824;INSUFFICIENT_OBS,NONE,0.000000000,0.000000000,0.000000000,0.0,0.000000000,0.000000000,\"\",0,0,0,0,00,00,00,00*fb3df011\n\tsystem status\tnormal 2 27.800000 0 0\trobot status\t299.129711\t58.993261\t10.364500\t0.469342\t3.019620\t-31.495891\t0.170000\t0.212000\n\t\n15:24:44.1\tlog_raw\tgps_raw\t#DUALANTENNAHEADINGA,USB3,0,49.0,FINESTEERING,2107,282302.100,02000000,d426,15824;SOL_COMPUTED,NARROW_FLOAT,-1.000000000,117.785400391,-42.761993408,0.0,360.000000000,180.000000000,\"631T\",16,6,6,5,04,00,20,03*f6212de6\n\tsystem status\tnormal 2 27.800000 0 0\trobot status\t299.245599\t58.913078\t10.369800\t0.415488\t2.908104\t-30.773651\t0.318000\t-0.017000\n\t\n15:24:44.6\tlog_raw\tgps_raw\t#INSPVAXA,USB3,0,51.5,FINESTEERING,2107,282302.600,02000000,471d,15824;INS_ALIGNMENT_COMPLETE,INS_RTKFIXED,37.37066035921,126.72421474502,10.3743,22.3000,-0.1596,0.2340,0.0126,0.411007245,2.764808403,120.160386775,0.5045,0.3294,0.6194,0.1239,0.0993,0.0801,0.1433,0.1477,4.9538,0f000001,0*7b8f0c3b\n\tsystem status\tnormal 2 27.900000 0 0\trobot status\t299.362969\t58.834535\t10.374300\t0.411007\t2.764808\t-30.160387\t0.179000\t0.195000\n\t\n15:24:45.1\tlog_raw\tgps_raw\t#DUALANTENNAHEADINGA,USB3,0,49.5,FINESTEERING,2107,282303.100,02000000,d426,15824;INSUFFICIENT_OBS,NONE,0.000000000,0.000000000,0.000000000,0.0,0.000000000,0.000000000,\"\",0,0,0,0,00,00,00,00*96d140e5\n\tsystem status\tnormal 2 27.900000 0 0\trobot status\t299.479291\t58.756826\t10.380500\t0.400362\t2.527135\t-29.573701\t0.341000\t-0.036000\n\t\n15:24:45.6\tlog_raw\tgps_raw\t#DUALANTENNAHEADINGA,USB3,0,49.5,FINESTEERING,2107,282303.600,02000000,d426,15824;INSUFFICIENT_OBS,NONE,0.000000000,0.000000000,0.000000000,0.0,0.000000000,0.000000000,\"\",0,0,0,0,00,00,00,00*3f9a20d4\n\tsystem status\tnormal 2 27.900000 0 0\trobot status\t299.591664\t58.676294\t10.392400\t0.413506\t2.330226\t-29.178083\t0.309000\t-0.008000\n\t\n15:24:46.1\tlog_raw\tgps_raw\t#INSPVAXA,USB3,0,43.0,FINESTEERING,2107,282304.100,02000000,471d,15824;INS_ALIGNMENT_COMPLETE,INS_RTKFIXED,37.37065823022,126.72421863146,10.4032,22.3000,-0.1537,0.2368,0.0051,0.137147576,2.044689982,118.905091584,0.5709,0.3745,0.6911,0.1341,0.1081,0.0826,0.1447,0.1492,4.9492,0f000001,0*2d96de96\n\tsystem status\tnormal 2 28.000000 0 0\trobot status\t299.707223\t58.598237\t10.403200\t0.137148\t2.044690\t-28.905092\t0.469000\t-0.234000\n\t\n15:24:46.6\tlog_raw\tgps_raw\t#DUALANTENNAHEADINGA,USB3,0,43.0,FINESTEERING,2107,282304.600,02000000,d426,15824;INSUFFICIENT_OBS,NONE,0.000000000,0.000000000,0.000000000,0.0,0.000000000,0.000000000,\"\",0,0,0,0,00,00,00,00*c23e1cc5\n\tsystem status\tnormal 2 28.000000 0 0\trobot status\t299.825380\t58.523361\t10.407700\t0.067712\t1.877475\t-28.805991\t0.317000\t-0.040000\n\t\n15:24:47.1\tlog_raw\tgps_raw\t#DUALANTENNAHEADINGA,USB3,0,43.0,FINESTEERING,2107,282305.100,02000000,d426,15824;SOL_COMPUTED,L1_FLOAT,-1.000000000,149.112899780,-55.880187988,0.0,360.000000000,180.000000000,\"631T\",16,6,6,5,04,00,20,03*c998c635\n\tsystem status\tnormal 2 28.000000 0 0\trobot status\t299.941727\t58.448647\t10.413200\t0.066472\t1.938799\t-28.796834\t0.304000\t-0.015000\n\t\n15:24:47.6\tlog_raw\tgps_raw\t#INSPVAXA,USB3,0,50.0,FINESTEERING,2107,282305.600,02000000,471d,15824;INS_ALIGNMENT_COMPLETE,INS_RTKFIXED,37.37065621091,126.72422257875,10.4180,22.3000,-0.1470,0.2285,0.0045,0.107072470,2.040461539,118.820220655,0.5709,0.3745,0.6911,0.1341,0.1081,0.0826,0.1447,0.1492,4.9492,0f000001,0*28a83c0b\n\tsystem status\tnormal 2 28.000000 0 0\trobot status\t300.056868\t58.374112\t10.418000\t0.107072\t2.040462\t-28.820221\t0.293000\t-0.011000\n\t\n15:24:48.1\tlog_raw\tgps_raw\t#DUALANTENNAHEADINGA,USB3,0,49.0,FINESTEERING,2107,282306.100,02000000,d426,15824;SOL_COMPUTED,NARROW_FLOAT,-1.000000000,131.179367065,-49.751617432,0.0,360.000000000,180.000000000,\"631T\",16,6,6,5,04,00,20,03*d544857e\n\tsystem status\tnormal 2 28.000000 0 0\trobot status\t300.170789\t58.298975\t10.424400\t-0.098983\t2.017315\t-28.907461\t0.301000\t-0.013000\n\t\n15:24:48.6\tlog_raw\tgps_raw\t#INSPVAXA,USB3,0,49.0,FINESTEERING,2107,282306.600,02000000,471d,15824;INS_ALIGNMENT_COMPLETE,INS_RTKFIXED,37.37065472577,126.72422510434,10.4346,22.3000,-0.1517,0.2382,0.0100,-0.069215248,2.129232392,118.969367736,0.5936,0.3892,0.7368,0.1380,0.1115,0.0828,0.1450,0.1498,4.9367,0f000001,0*a2c53eca\n\tsystem status\tnormal 2 28.100000 0 0\trobot status\t300.280580\t58.209277\t10.434600\t-0.069215\t2.129232\t-28.969368\t0.298000\t-0.019000\n\t\n15:24:49.1\tlog_raw\tgps_raw\t#DUALANTENNAHEADINGA,USB3,0,48.0,FINESTEERING,2107,282307.100,02000000,d426,15824;INSUFFICIENT_OBS,NONE,0.000000000,0.000000000,0.000000000,0.0,0.000000000,0.000000000,\"\",0,0,0,0,00,00,00,00*83621ed4\n\tsystem status\tnormal 2 28.000000 0 0\trobot status\t300.390113\t58.121203\t10.443900\t0.002620\t2.258419\t-29.033865\t0.296000\t-0.022000\n\t\n15:24:49.6\tlog_raw\tgps_raw\t#DUALANTENNAHEADINGA,USB3,0,48.0,FINESTEERING,2107,282307.600,02000000,d426,15824;INSUFFICIENT_OBS,NONE,0.000000000,0.000000000,0.000000000,0.0,0.000000000,0.000000000,\"\",0,0,0,0,00,00,00,00*2a297ee5\n\tsystem status\tnormal 2 28.000000 0 0\trobot status\t300.507756\t58.037733\t10.451400\t-0.138265\t2.169537\t-29.248611\t0.307000\t-0.015000\n\t\n15:24:50.1\tlog_raw\tgps_raw\t#DUALANTENNAHEADINGA,USB3,0,48.0,FINESTEERING,2107,282308.100,02000000,d426,15824;SOL_COMPUTED,NARROW_FLOAT,-1.000000000,130.346817017,-46.744110107,0.0,360.000000000,180.000000000,\"631T\",13,6,6,5,04,00,20,03*2381209c\n\tsystem status\tnormal 2 28.000000 0 0\trobot status\t300.624124\t57.953181\t10.459000\t-0.080072\t2.139978\t-29.443708\t0.298000\t-0.017000\n\t\n15:24:50.6\tlog_raw\tgps_raw\t#DUALANTENNAHEADINGA,USB3,0,50.0,FINESTEERING,2107,282308.600,02000000,d426,15824;SOL_COMPUTED,NARROW_FLOAT,-1.000000000,131.524536133,-48.144073486,0.0,360.000000000,180.000000000,\"631T\",17,6,6,5,04,00,20,03*26d8279d\n
